vi "画矩形2.vi"(10 "新矩形":dbl[](array[numeric]), 11 "引用句柄输入":T1) -> ()   [LabVIEW 2014]
uses:
  <vilib>/vision/Image Controls.llb/IMAQ Image.ctl
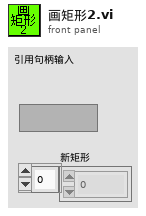
[diagram p1: front panel]
types:
  T1 = typedef "IMAQ Image.ctl" = refnum<image>
  T2 = cluster{"新矩形[0]":dbl, "新矩形[1]":dbl, "新矩形[2]":dbl, "新矩形[3]":dbl}
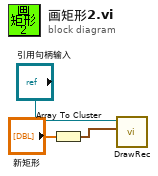
[diagram p0: block diagram]
diagram:
  n1 = Array To Cluster(array="新矩形") -> (cluster=w1:T2)
  n2 = call "DrawRec.vi"("Rectangle"=w1, "Image"="引用句柄输入") -> ()  [unwired: 9 in, 1 out]
